vi "Set System Resources.vi"(8 "error in (no error)":errorcluster) -> (0 "error out":errorcluster)   [LabVIEW 2020]
doc: "This VI gets the system session and system reference and puts it on the appropriate notifier."
uses:
  Type Definitions/System Resources.ctl
  <vilib>/FPGAPlugInAG/sbRIO-9651/niLvFpga_Open_sbRIO-9651.vi
  <vilib>/rvi/interface/common/dynamic/niFpgaDynamicAddResources.vi
  <vilib>/FPGAPlugInAG/Dynamic/niLvFpga_Reset_Dynamic.vi
  <vilib>/FPGAPlugInAG/Dynamic/niLvFpga_Run_Dynamic.vi
  <vilib>/rvi/interface/nirviOpenFPGA/nirviOpenFPGA.xnode
  Phantom/Avionics Software/Projects/Alterrum.git/trunk/Embedded Core/Builds/FPGA Bitfiles/FPGA_Main.lvbitx
  <vilib>/rvi/interface/nirviMethod/nirviMethod.xnode
  <vilib>/nisyscfg/nisyscfg.lvlib
  <resource>/objmgr/nisysapi.rc
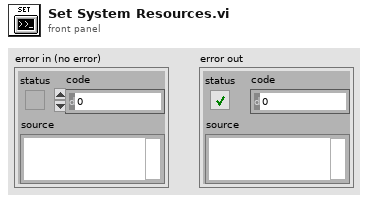
[diagram p1: front panel]
types:
  T1 = typedef "System Resources.ctl" = cluster{"System Session":refnum<k21>, "System Resource":refnum<k20>, "FPGA VI Reference":refnum<k20>}
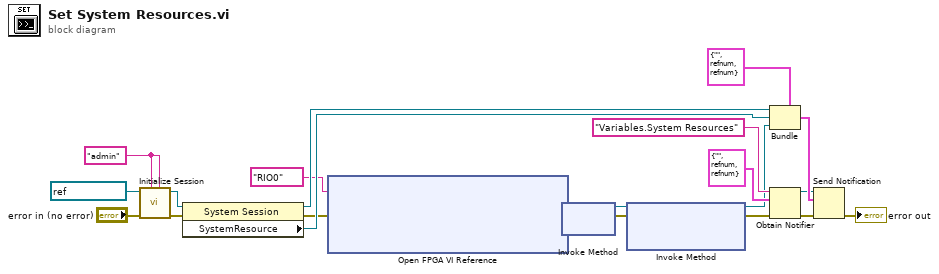
[diagram p0: block diagram]
diagram:
  w9 = "admin" ("User Name")
  n1 = call <vilib>:"Initialize Session.vi"("Password"=w9, "User Name"=w9, "error in (no error)"="error in (no error)", "Target (localhost)"=refnum<k21> "localhost") -> ("error out"=w11:errorcluster, "Session out"=w10:refnum<k21>)  [unwired: 6 in]
  n2 = property class="System Session"(reference=w10, error in=w11) -> (reference out=w13:refnum<k21>, error out=w7:errorcluster, "SystemResource"=w14:refnum<k20>)
  n3 = xnode "Open FPGA VI Reference"("error in"=w7, "resource name"=tag "RIO0") -> ("FPGA VI Reference Out"=w5:refnum<k20>, "error out"=w6:errorcluster)
  n4 = xnode "Invoke Method"("FPGA VI Reference In"=w5, "error in"=w6) -> ("FPGA VI Reference Out"=w2:refnum<k20>, "error out"=w4:errorcluster)
  n5 = xnode "Invoke Method"("FPGA VI Reference In"=w2, "error in"=w4) -> ("FPGA VI Reference Out"=w1:refnum<k20>, "error out"=w3:errorcluster)  [unwired: 1 in]
  n6 = Bundle(cluster=T1 {"System Session"="", "System Resource"=refnum, "FPGA VI Reference"=refnum}, "System Session"=w13, "System Resource"=w14, "FPGA VI Reference"=w1) -> (w19:T1)
  n7 = Obtain Notifier(name (unnamed)="Variables.System Resources", notification data type=T1 {"System Session"="", "System Resource"=refnum, "FPGA VI Reference"=refnum} ("cluster"), error in (no error)=w3) -> (notifier out=w18:refnum<notifier>, error out=w21:errorcluster)  [unwired: 1 in, 1 out]
  n8 = Send Notification(notification=w19, notifier=w18, error in (no error)=w21) -> (error out=→"error out":errorcluster)  [unwired: 1 out]
